vi "To Hokuyo Data.vi"(9 "String Characters":string="VV", 10 "Serial Command":string="VV") -> (2 "Command String":string)   [LabVIEW 2018]
doc: "This VI takes a <b>Serial Command</b> and <b>String Characters</b> inputs and produces a <b>Command String</b> in a compatible form for the URG-04LX-UG01 to respond to. \n\n<b>Serial Command</b> and <b>String Characters</b> combinations can be found in the device datasheet."
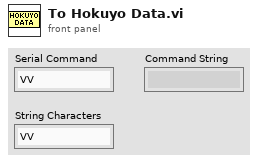
[diagram p1: front panel]
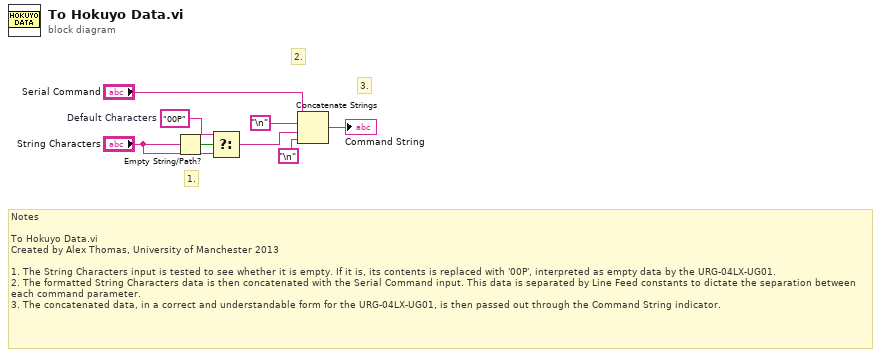
[diagram p0: block diagram]
diagram:
  w5 = "00P"  # Default Characters
  # "Notes\n\nTo Hokuyo Data.vi\nCreated by Alex Thomas, University of Manchester 2013\n\n1. The String Characters input is tested to see whether it is empty. If it is, its contents is replaced with '00P', interpreted as empty data by the URG-04LX-UG01.\n2. The formatted String Characters data is then concatenated with the Serial Command input. This data is separated by Line Feed constants to dictate the separation between each command parameter.\n3. The concatenated data, in a correct and understandable form for the URG-04LX-UG01, is then passed out through the Command String indicator."
  # "3."
  # "2."
  # "1."
  n1 = Empty String/Path?(string/path="String Characters") -> (empty?=w3:bool)
  n2 = Select(t=w5, s=w3, f="String Characters") -> (s? t:f=w6:string)
  n3 = Concatenate Strings("Serial Command", "\n", w6, "\n") -> (→"Command String":string)
